vi "Configure Digital Input Phase Noise.vi"(6 "Level Amplitude (-7.00000000E+001 dBc/Hz)":dbl=-23.5 format="%.8e", 7 "Phase Noise Stop Frequency (3.00000000E+4 Hz)":dbl=30000.0 format="%.8e", 8 "error in (no error)":errorcluster, 9 "Phase Noise Start Frequency (1.00000000E+3 Hz)":dbl=1000.0 format="%.8e", 10 "Enable Phase Noise (F: Disable)":bool, 11 "VISA resource name":refnum<visa-resource-name>) -> (0 "error out":errorcluster, 3 "VISA resource name out":refnum<visa-resource-name>)   [LabVIEW 2018, in "Agilent PSG MXG Series.lvlib"]
doc: "Configures the digital input phase noise settings.\n\n<b>Note:</b>\nIt is applicable for N5172B/82B with <b>Option 004</b> only."
uses:
  Agilent PSG MXG Series.lvlib
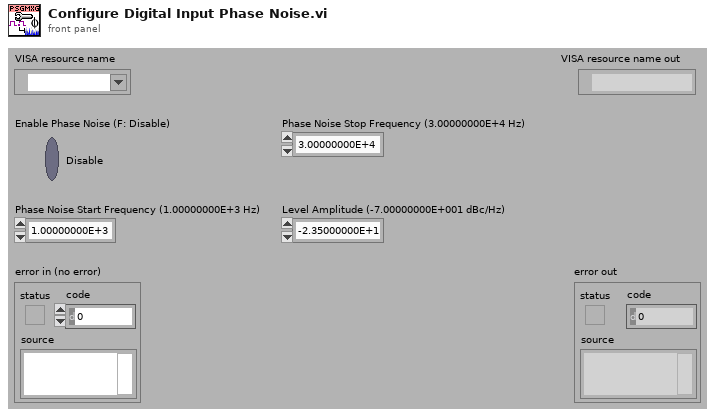
[diagram p1: front panel]
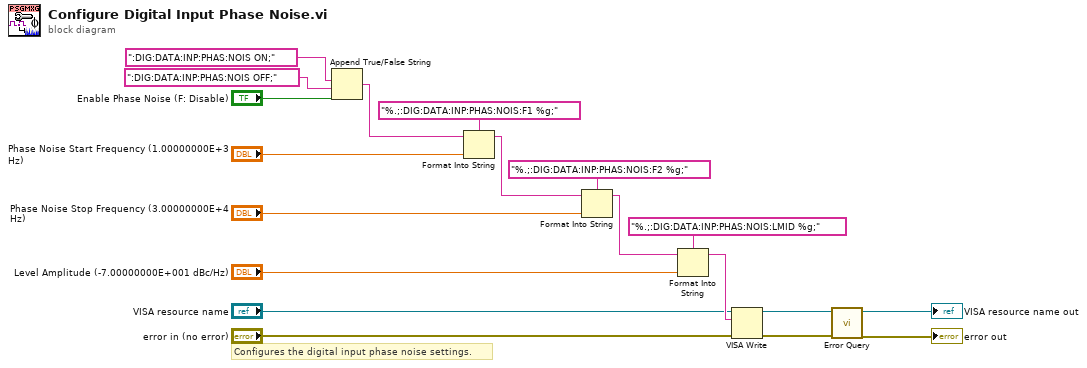
[diagram p0: block diagram]
diagram:
  # "Configures the digital input phase noise settings."
  n1 = Append True/False String(1:"Enable Phase Noise (F: Disable)", 2:":DIG:DATA:INP:PHAS:NOIS OFF;", 3:":DIG:DATA:INP:PHAS:NOIS ON;") -> (0:w16:string)  [unwired: 1 in]
  n2 = Format Into String(format string="%.;:DIG:DATA:INP:PHAS:NOIS:F1 %g;", initial string=w16, "Phase Noise Start Frequency (1.00000000E+3 Hz)") -> (resulting string=w13:string)  [unwired: 1 in, 1 out]
  n3 = Format Into String(format string="%.;:DIG:DATA:INP:PHAS:NOIS:F2 %g;", initial string=w13, "Phase Noise Stop Frequency (3.00000000E+4 Hz)") -> (resulting string=w10:string)  [unwired: 1 in, 1 out]
  n4 = Format Into String(format string="%.;:DIG:DATA:INP:PHAS:NOIS:LMID %g;", initial string=w10, "Level Amplitude (-7.00000000E+001 dBc/Hz)") -> (resulting string=w7:string)  [unwired: 1 in, 1 out]
  n5 = VISA Write(VISA resource name="VISA resource name", write buffer=w7, error in (no error)="error in (no error)") -> (VISA resource name out=w4:refnum<visa-resource-name>, error out=w3:errorcluster)  [unwired: 1 out]
  n6 = call "Error Query.vi"("error in (no error)"=w3, "VISA resource name"=w4) -> ("error out"=→"error out":errorcluster, "VISA resource name out"=→"VISA resource name out":refnum<visa-resource-name>)  [unwired: 6 in, 2 out]
